vi "IDS_select_IP_pop_up.vi"(10 "IPs":string[](array[string]), 11 "Found Devices":T1(array[cluster])) -> (2 "Device Info":T2, 3 "IP":string)   [LabVIEW 2016]
panel:
  out "error out":errorcluster
  out "Found devices":i32
  in  "please select IP":u16(ring) items=["10.10.1.122", "10.10.1.167", "10.10.1.196", "192.168.1.1"]
  in  "Refresh Button":bool
  in  "Process Stop":bool
  in  "OK Button":bool
  out "Array":T1(array[cluster])
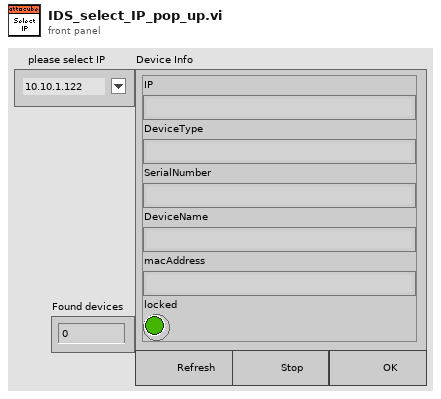
[diagram p1: front panel]
types:
  T1 = cluster{"IP":string, "DeviceType":string, "SerialNumber":string, "DeviceName":string, "macAddress":string, "locked":bool}[]
  T2 = cluster{"IP":string, "DeviceType":string, "SerialNumber":string, "DeviceName":string, "macAddress":string, "locked":bool}
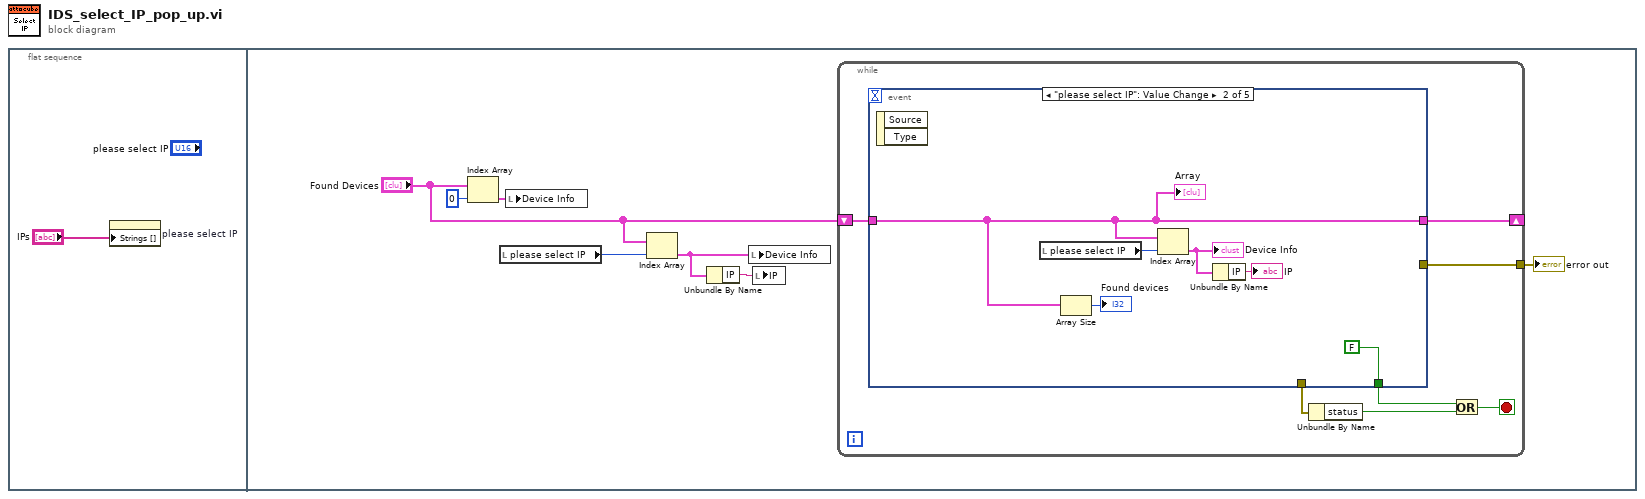
[diagram p0: block diagram]
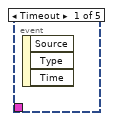
[diagram p2: hidden frame]
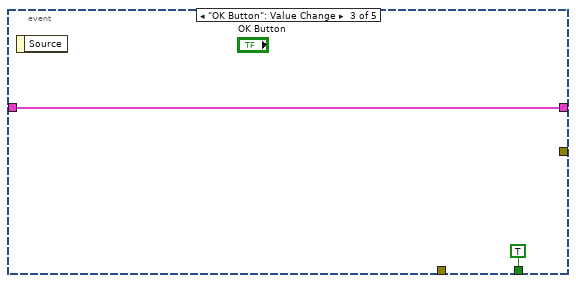
[diagram p3: hidden frame]
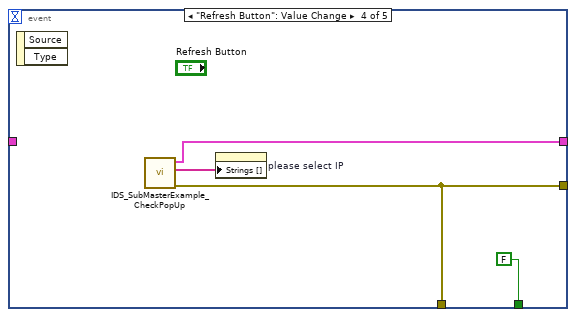
[diagram p4: hidden frame]
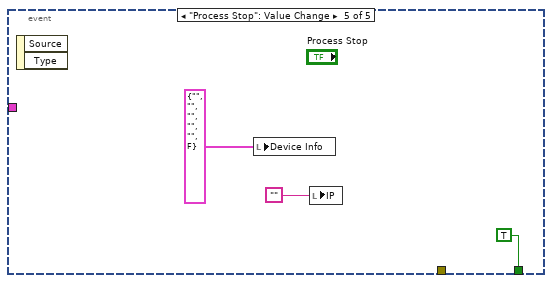
[diagram p5: hidden frame]
diagram:
  n1 = flat-sequence {
    frame #0 {
      n2 = property on="please select IP" class="Ring (strict)"("Strings []"="IPs") -> ()  [unwired: 2 in, 2 out]
    }
    frame #1 {
      n3 = Index Array(array="Found Devices", index=0) -> (element=w6:T2)
      n4 = local read "please select IP"() -> (w2:u16)
      n5 = local write "Device Info"(w6) -> ()
      n6 = Index Array(array="Found Devices", index=w2) -> (element=w3:T2)
      n7 = Unbundle By Name(w3) -> ("IP"=w4:string)
      n8 = local write "Device Info"(w3) -> ()
      n9 = local write "IP"(w4) -> ()
      n10 = while {
        shift-right: [w15] -> _
        shift-left: "Found Devices" -> [w9]
        tunnel: [w10] -> w8
        stop <- w11 stop-if-true
        n11 = event shown="[1] \"please select IP\": Value Change" {
          selector: _ -> [_ _ _ _ _]
          dyn-events: _ -> [_ _ _ _ _]
          timeout: _ -> [_ _ _ _ _]
          tunnel: [_ w19 w23 w27 _] -> w15
          tunnel: w9 -> [_ w19 w23 _ _]
          tunnel: [_ FALSE TRUE FALSE TRUE] -> w13
          tunnel: [_ _ _ w25 _] -> w14
          tunnel: [_ _ _ w25 _] -> w10
          event Timeout {
            n12 = event-data() -> ()  [unwired: 1 in, 3 out]
          }
          event "please select IP": Value Change {
            n13 = event-data() -> ()  [unwired: 1 in, 2 out]
            n14 = local read "please select IP"() -> (w16:u16)
            n15 = Array Size(array=w19) -> (size(s)=→"Found devices":i32)
            n16 = Index Array(array=w19, index=w16) -> (element=w18:T2)
            "Device Info" <- w18
            n17 = Unbundle By Name(w18) -> ("IP"=→"IP":string)
            "Array" <- w19
          }
          event "OK Button": Value Change {
            n18 = event-data() -> ()  [unwired: 1 in, 1 out]
          }
          event "Refresh Button": Value Change {
            n19 = event-data() -> ()  [unwired: 1 in, 2 out]
            n20 = call "IDS_SubMasterExample_CheckPopUp.vi"() -> ("error out"=w25:errorcluster, "IPs"=w24:string[], "Found Devices"=w27:T1)  [unwired: 8 in, 1 out]
            n21 = property on="please select IP" class="Ring (strict)"("Strings []"=w24) -> ()  [unwired: 2 in, 2 out]
          }
          event "Process Stop": Value Change {
            n22 = event-data() -> ()  [unwired: 1 in, 2 out]
            n23 = local write "Device Info"(T2 {"IP"="", "DeviceType"="", "SerialNumber"="", "DeviceName"="", "macAddress"="", "locked"=FALSE} ("Cluster")) -> ()
            n24 = local write "IP"("") -> ()
          }
        }
        n25 = Unbundle By Name(w14) -> ("status"=w12:bool)
        n26 = Or(x=w13, y=w12) -> (x .or. y?=w11:bool)
      }
      "error out" <- w8
    }
  }
